vi "Read Check Revocation.vi"(8 "error in (no error)":errorcluster, 11 "dotNET SSL Server in":refnum<class "dotNET SSL Socket.lvclass">) -> (0 "error out":errorcluster, 2 "Check Revocation":bool, 3 "dotNET SSL Server out":refnum<class "dotNET SSL Socket.lvclass">)   [LabVIEW 2013, in "dotNET SSL Socket.lvlib" / "dotNET SSL Socket.lvclass"]
uses:
  dotNET SSL Socket.lvclass
  dotNET SSL Socket.lvclass/dotNET SSL Socket.ctl
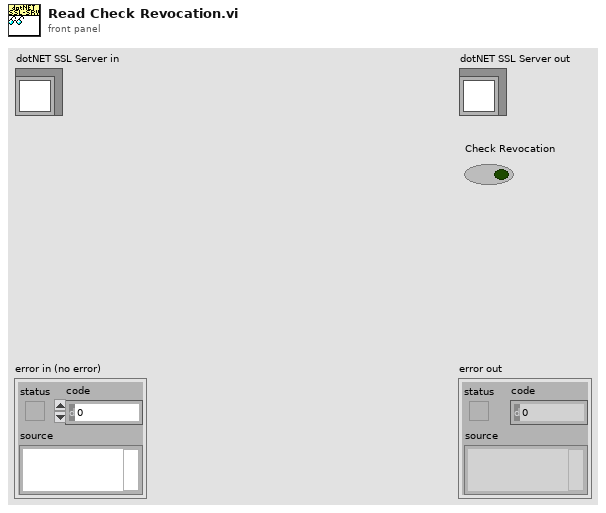
[diagram p1: front panel]
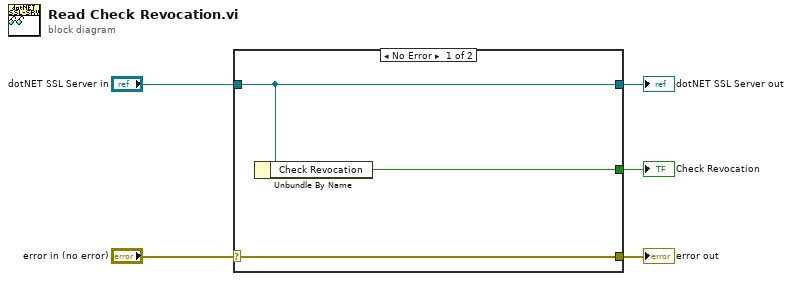
[diagram p0: block diagram]
diagram:
  n1 = case shown="No Error" "error in (no error)" {
    selector: "error in (no error)" -> [w8 w9]
    tunnel: [w8 w9] -> w4
    tunnel: [w7 w10] -> w2
    tunnel: "dotNET SSL Server in" -> [w7 w10]
    tunnel: [w6 _] -> w1
    frame No Error {
      n2 = Unbundle By Name(w7) -> ("Check Revocation"=w6:bool)
    }
    frame Error {
    }
  }
  "error out" <- w4
  "dotNET SSL Server out" <- w2
  "Check Revocation" <- w1
